vi "Custom Message.vi"(6 "Boolean Text":string="OK", 7 "MSG":string) -> ()   [LabVIEW 2021]
panel:
  in  "OK":bool
  in  "Title":string
  out "Ok?":bool
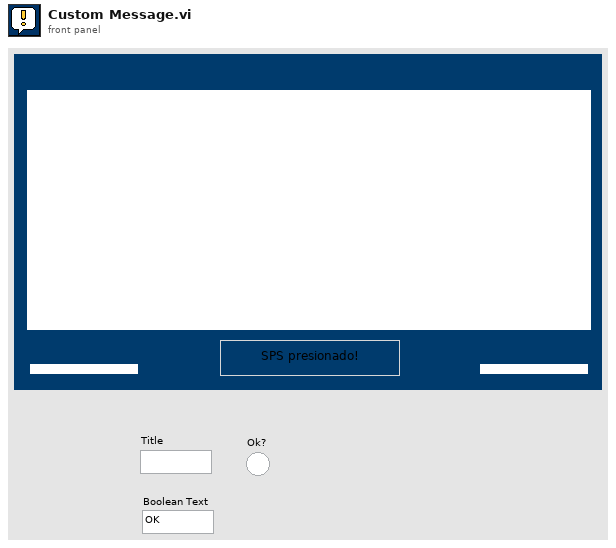
[diagram p1: front panel]
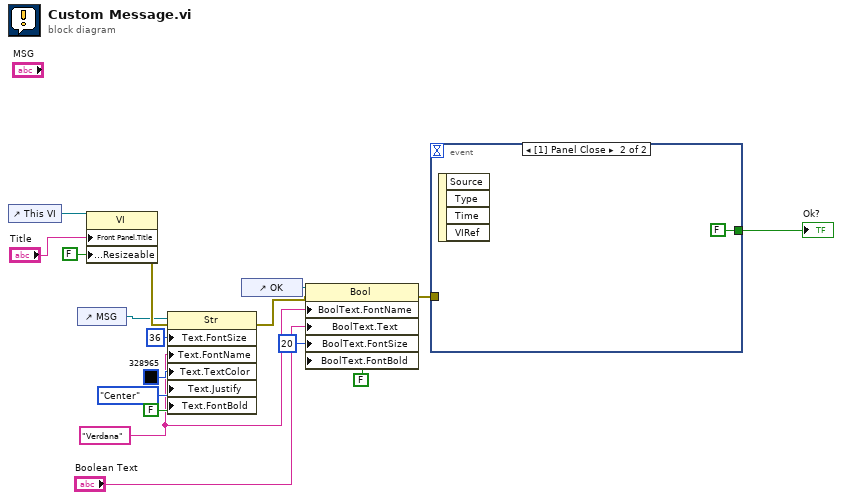
[diagram p0: block diagram]
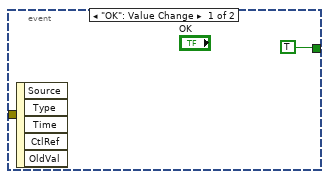
[diagram p2: hidden frame]
diagram:
  w4 = "Verdana" ("Text.Font:Name")
  n1 = control-ref of="This VI"() -> (w13:refnum<vi>)
  n2 = control-ref of="MSG"() -> (w5:refnum<vi>)
  n3 = property class="VI"(reference=w13, "Front Panel.Title"="Title", "Front Panel.Resizeable"=FALSE ("Front Panel Window:Resizable")) -> (error out=w11:errorcluster)  [unwired: 1 in, 1 out]
  n4 = property on="Property Node" class="Str"(reference=w5, error in=w11, "Text.FontSize"=u32 36 ("Text.Font:Size"), "Text.FontName"=w4, "Text.TextColor"=u32 328965 ("Text.Text Colors:Text Color"), "Text.Justify"=enum16{"Left", "Center", "Right"}."Center" ("Text.Justification"), "Text.FontBold"=FALSE ("Text.Font:Bold")) -> (error out=w7:errorcluster)  [unwired: 1 out]
  n5 = control-ref of="OK"() -> (w8:refnum<vi>)
  n6 = property on="Property Node" class="Bool"(reference=w8, error in=w7, "BoolText.FontName"=w4, "BoolText.Text"="Boolean Text", "BoolText.FontSize"=u32 20 ("Boolean Text.Font:Size"), "BoolText.FontBold"=FALSE ("Boolean Text.Font:Bold")) -> (error out=w6:errorcluster)  [unwired: 1 out]
  n7 = event shown="[1] Panel Close" {
    selector: _ -> [_ _]
    dyn-events: _ -> [_ _]
    timeout: _ -> [_ _]
    tunnel: [TRUE FALSE] -> w14
    tunnel: w6 -> [_ _]
    event "OK": Value Change {
      n8 = event-data() -> ()  [unwired: 6 out]
    }
    event Panel Close {
      n9 = event-data() -> ()  [unwired: 5 out]
    }
  }
  "Ok?" <- w14
